vi "edittest save step.vi"(8 "error in (no error)":errorcluster, 9 "POST (empty)":T3, 10 "sxSequenceId (\"\")":string, 11 "Connection Refnum":T2) -> (0 "error out":errorcluster, 2 "New Step Record":T1, 3 "Connection Refnum":T2)   [LabVIEW 2011]
uses:
  Addons/internet/utils/keyedarr.llb/Keyed Array.ctl
  SI.LIB/ODBC/SQL Controls/Connection Refnum.ctl
  server/database/Steps/Step Record.ctl
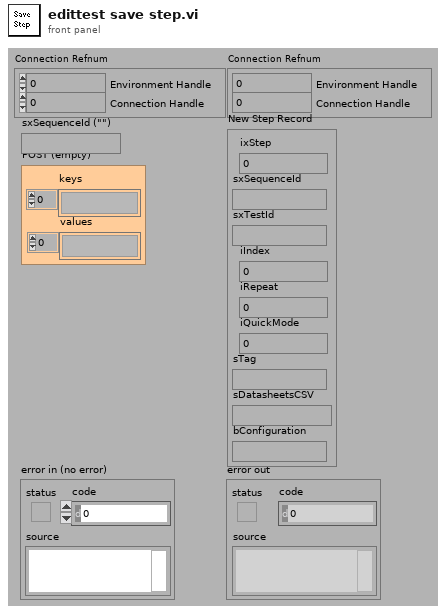
[diagram p1: front panel]
types:
  T1 = typedef "Step Record.ctl" = cluster{"ixStep":i32, "sxSequenceId":string, "sxTestId":string, "iIndex":i32, "iRepeat":i32, "iQuickMode":i32, "sTag":string, "sDatasheetsCSV":string, "bConfiguration":string}
  T2 = typedef "Connection Refnum.ctl" = cluster{"Environment Handle":i32, "Connection Handle":i32}
  T3 = typedef "Keyed Array.ctl" = cluster{"keys":string[], "values":string[]}
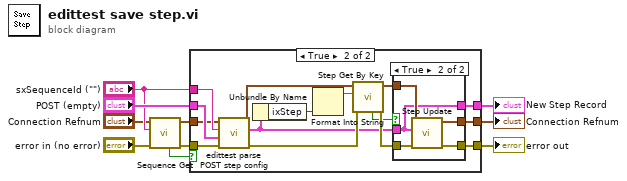
[diagram p0: block diagram]
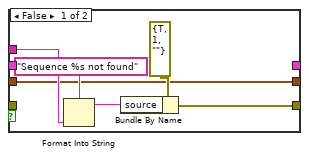
[diagram p2: hidden frame]
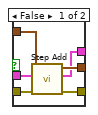
[diagram p3: hidden frame]
diagram:
  n1 = call "Sequence Get.vi"("error in (no error)"="error in (no error)", "sxSequenceId (\"\")"="sxSequenceId (\"\")", "Connection Refnum"="Connection Refnum") -> ("error out"=w7:errorcluster, "Connection Refnum"=w2:T2, "Data Present"=w6:bool)  [unwired: 6 out]
  n2 = case shown="True" w6 {
    tunnel: [w13 w31] -> w10
    tunnel: "POST (empty)" -> [_ w28]
    tunnel: w7 -> [_ w30]
    tunnel: "sxSequenceId (\"\")" -> [w15 w27]
    tunnel: [w11 w29] -> w4
    tunnel: w2 -> [w11 w26]
    tunnel: [_ w17] -> w1
    frame False {
      n3 = Format Into String(format string="Sequence %s not found" ("source"), w15) -> (resulting string=w12:string)  [unwired: 2 in, 1 out]
      n4 = Bundle By Name(cluster=errorcluster {"status"=TRUE, "code"=1, "source"=""} ("error out"), "source"=w12) -> (w13:errorcluster)
    }
    frame True {
      n5 = call "edittest parse POST step config.vi"("error in (no error)"=w30, "POST (empty)"=w28, "sxSequenceId (\"\")"=w27, "Connection Refnum"=w26) -> ("error out"=w25:errorcluster, "Step Record"=w21:T1, "dup Connection Refnum"=w24:T2)  [unwired: 5 out]
      n6 = Unbundle By Name(w21) -> ("ixStep"=w20:i32)
      n7 = Format Into String(w20) -> (resulting string=w19:string)  [unwired: 3 in, 1 out]
      n8 = call "Step Get By Key.vi"("error in (no error)"=w25, "ixStep"=w19, "Connection Refnum"=w24) -> ("error out"=w22:errorcluster, "Connection Refnum"=w23:T2, "Data Present"=w18:bool)  [unwired: 5 in, 1 out]
      n9 = case shown="True" w18 {
        tunnel: [w37 w42] -> w31
        tunnel: [w36 w41] -> w29
        tunnel: w23 -> [w35 w40]
        tunnel: w22 -> [w34 w39]
        tunnel: w21 -> [w33 w38]
        tunnel: [w32 w38] -> w17
        frame False {
          n10 = call "Step Add.vi"("error in (no error)"=w34, "Step Record"=w33, "Connection Refnum"=w35) -> ("error out"=w37:errorcluster, "New Step Record"=w32:T1, "Connection Refnum"=w36:T2)  [unwired: 6 out]
        }
        frame True {
          n11 = call "Step Update.vi"("error in (no error)"=w39, "Step Record (empty)"=w38, "Connection Refnum"=w40) -> ("error out"=w42:errorcluster, "Connection Refnum"=w41:T2)  [unwired: 7 in]
        }
      }
    }
  }
  "error out" <- w10
  "Connection Refnum" <- w4
  "New Step Record" <- w1
